vi "Channel to Register.vi"(11 "Channel":T1) -> (3 "f":T2 items=["IODIRA"=0, "IODIRB"=1, "GPIOA"=18, "GPIOB"=19])   [LabVIEW 2020, in "MCP23017.lvclass"]
uses:
  MCP23017.lvclass
  Registers.ctl
  GPIO Channel.ctl
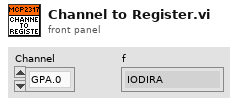
[diagram p1: front panel]
types:
  T1 = typedef "GPIO Channel.ctl" = enum16{"GPA.0", "GPA.1", "GPA.2", "GPA.3", "GPA.4", "GPA.5", "GPA.6", "GPA.7", "GPB.0", "GPB.1", "GPB.2", "GPB.3", "GPB.4", "GPB.5", "GPB.6", "GPB.7"}
  T2 = typedef "MCP23017.lvclass/Registers.ctl" = u16
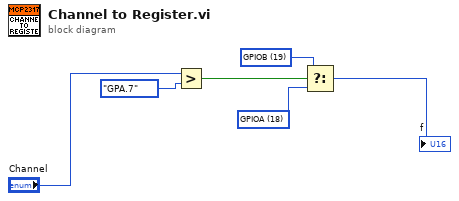
[diagram p0: block diagram]
diagram:
  w5 = T2 18 items=["IODIRA"=0, "IODIRB"=1, "GPIOA"=18, "GPIOB"=19] ("f")
  w1 = T2 19 items=["IODIRA"=0, "IODIRB"=1, "GPIOA"=18, "GPIOB"=19] ("Registers")
  n1 = Greater?(x="Channel", y=GPIO_Channel."GPA.7" ("Channel")) -> (0:w6:bool)
  n2 = Select(t=w1, s=w6, f=w5) -> (s? t:f=→"f":T2)
